vi "Shutdown Generator.vi"(8 "error in":errorcluster, 11 "next start sample":dbl) -> (0 "error out":errorcluster, 3 "total samples":dbl)   [LabVIEW 2026, in "Signal Generator.lvlib"]
doc: "Shutdown stage. Finalises a generation run when the client cancels or an error stops the acquisition loop and reports the total number of samples produced. The simulator holds no hardware sessions, files or other resources, so nothing needs to be closed here; this is the single place to release resources if the engine ever acquires any."
uses:
  Signal Generator.lvlib
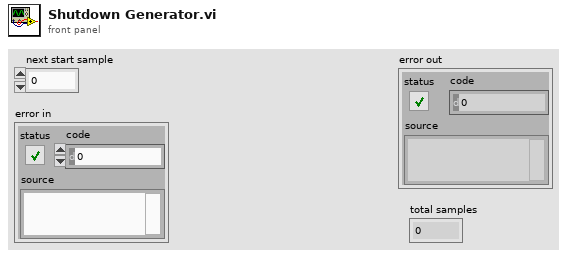
[diagram p1: front panel]
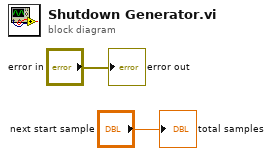
[diagram p0: block diagram]
diagram:
  "error out" <- "error in"
  "total samples" <- "next start sample"
